vi "next chunk - read-write freq PID file -analysis.vi"(4 "frequency":dbl, 6 "temperature":dbl format="%#_8g", 7 "PID action":T2, 8 "freq PID file OUT":string="peak_PID_scratch.dat", 9 "freq PID file IN":string="peak_PID.dat", 10 "PID freq IN":dbl[](array[numeric]), 11 "sweep folder path":path) -> (0 "temperatures":dbl[](array[numeric]), 1 "frequencies":dbl[][](array[numeric]), 2 "PID freq":dbl[](array[numeric]), 3 "sweep folder path out":path)   [LabVIEW 2012]
uses:
  next chunk read-write PID -- action.ctl
  ctl -- name dispatcher -- action.ctl
  file -- 9w path.vi
  array -- find index - real.vi
  array -- interpolate -- i.vi
  ctl -- name dispatcher.vi
  Q -- check range -- i -- real.vi
  Q - not nan -- real.vi
  <vilib>/Utility/libraryn.llb/Check if File or Folder Exists.vi
  file -- read list of lines.vi
  parse -- find first line.vi
  parse -- get list of matches -- numbers.vi
  <vilib>/Utility/file.llb/Write To Spreadsheet File.vi
  <vilib>/Utility/file.llb/Write To Spreadsheet File (string).vi
panel:
  in  "ctl kind IN":T1
  in  "ctl kind OUT":T1
  out "header":string[](array[string])
  out "number":i32=9
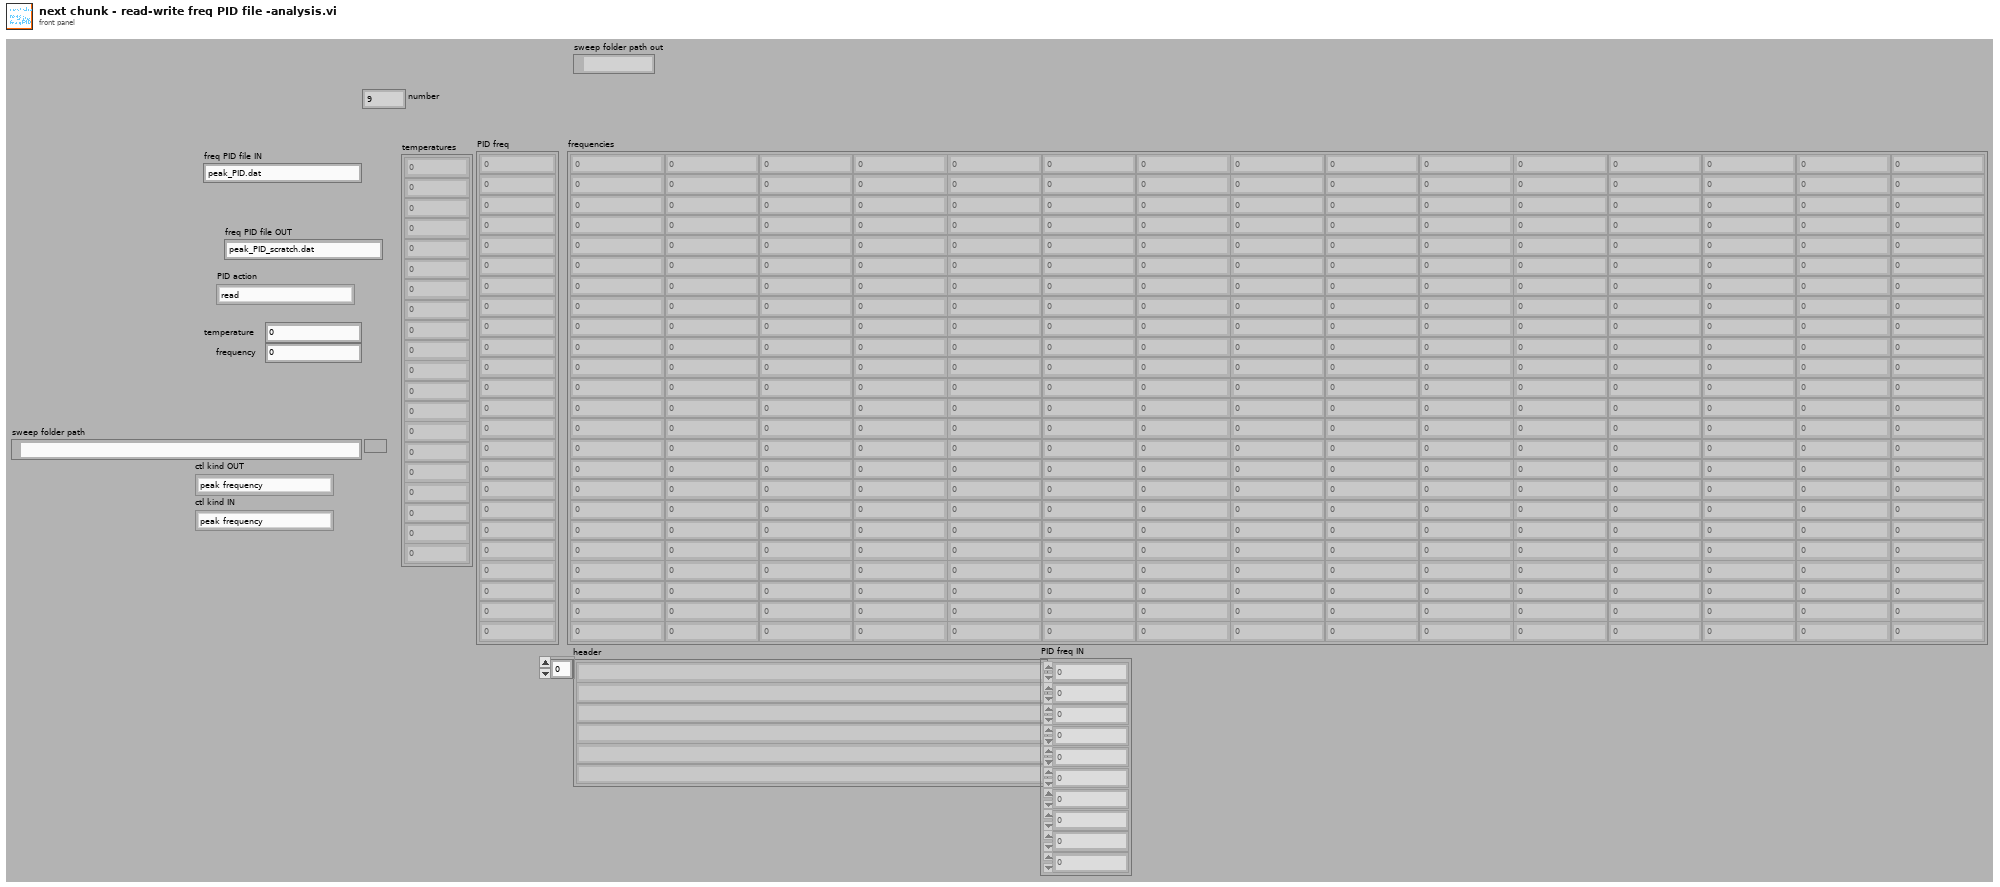
[diagram p1: front panel]
types:
  T1 = typedef "ctl -- name dispatcher -- action.ctl" = enum16{"peak frequency", "peak frequency DUMP", "peak gamma DUMP", "peak gamma", "peak frequency TEST", "peak gamma TEST", "ultrasonic power", "time in gamma", "set temperature ", "set temperature timer", "peak default gamma", "last scan file", "peak freq gamma TEST", "peak NAMES", "errors", "P_I_D", "P", "I", "D"}
  T2 = typedef "next chunk read-write PID -- action.ctl" = enum16{"read", "interpolate", "append col", "write", "write PID col", "append PID col", "interpolate - bezier"}
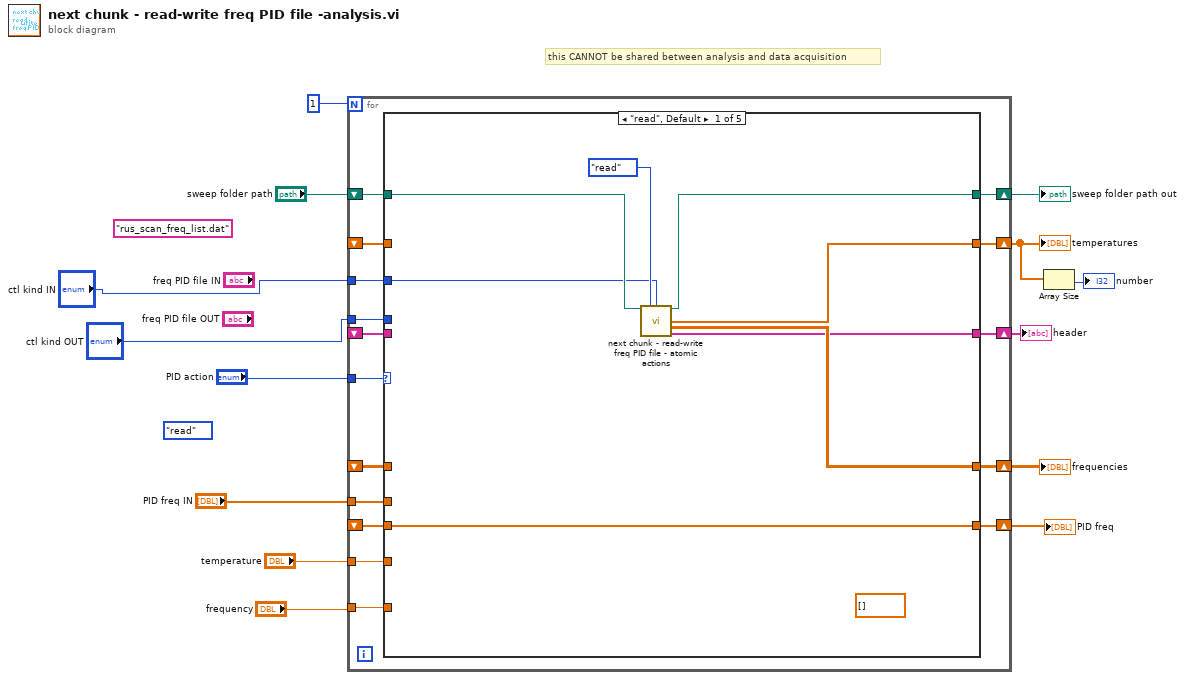
[diagram p0: block diagram]
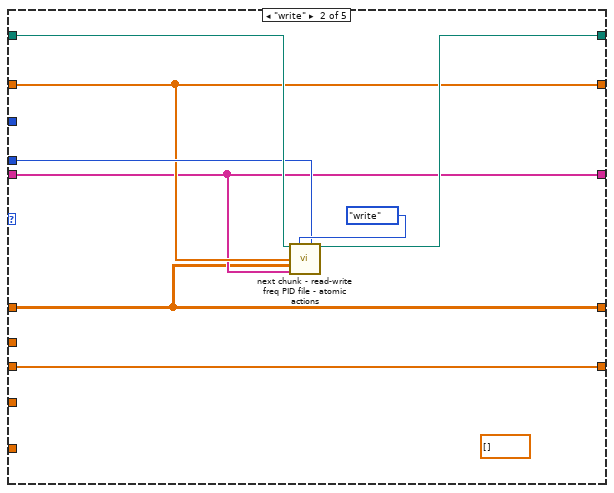
[diagram p2: hidden frame]
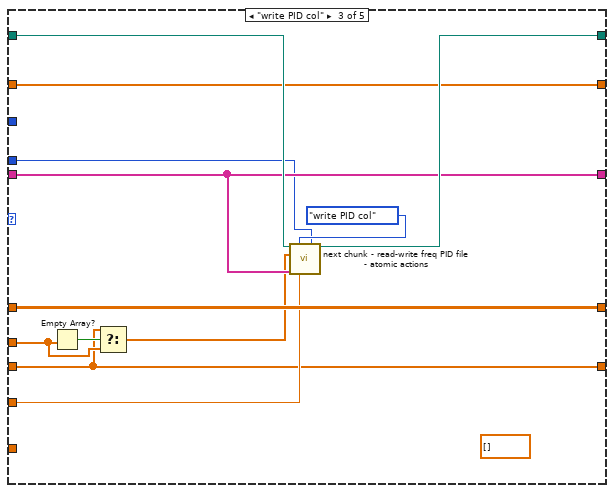
[diagram p3: hidden frame]
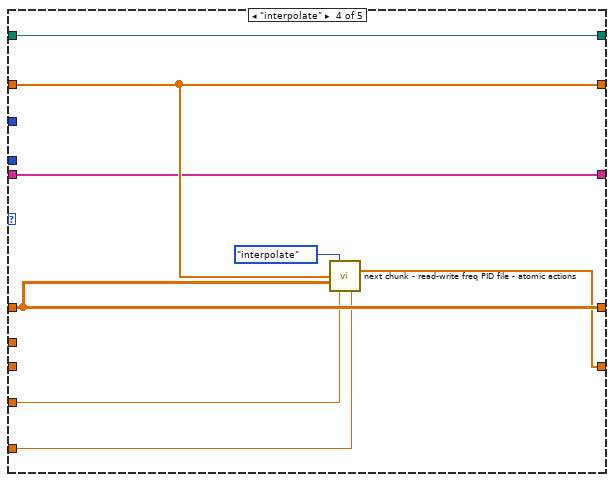
[diagram p4: hidden frame]
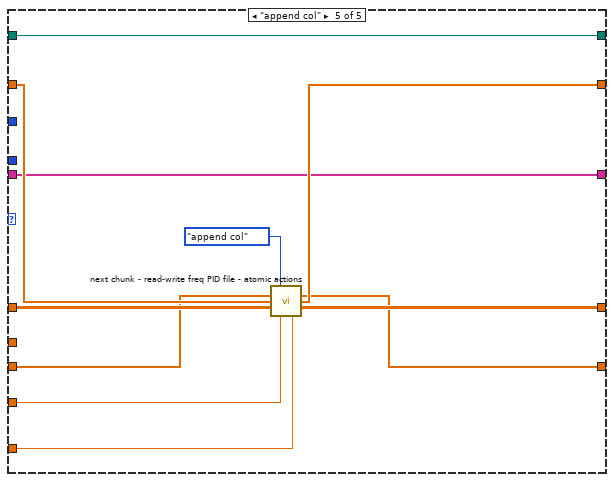
[diagram p5: hidden frame]
diagram:
  (unwired) next_chunk_read-write_PID_--_action."read" ("PID action")
  (unwired) "rus_scan_freq_list.dat" ("delimiter (\\t)")
  # "this CANNOT be shared between analysis and data acquisition"
  n1 = for {
    N: 1 -> [_]
    tunnel: "temperature" -> [w29]
    tunnel: "ctl kind IN" -> [w26]
    tunnel: "PID action" -> [w24]
    shift-right: [w30] -> w5
    shift-left: _ -> [w22]
    shift-right: [w25] -> w9
    shift-left: _ -> [w23]
    shift-right: [w28] -> w13
    shift-left: _ -> [w21]
    tunnel: "ctl kind OUT" -> [w20]
    tunnel: "frequency" -> [w19]
    shift-right: [w18] -> w6
    shift-left: "sweep folder path" -> [w27]
    shift-right: [w17] -> w4
    shift-left: _ -> [w16]
    tunnel: "PID freq IN" -> [w15]
    n2 = case shown="\"read\", Default" w24 {
      tunnel: [w34 w39 w53 w63 w73] -> w30
      tunnel: w29 -> [_ _ w52 w61 w71]
      tunnel: [w38 w46 w49 w62 w67] -> w28
      tunnel: w27 -> [w37 w45 w58 w66 w77]
      tunnel: w26 -> [w32 _ _ _ _]
      tunnel: [w33 w41 w55 w64 w72] -> w25
      tunnel: w23 -> [_ w41 w55 w64 w75]
      tunnel: w22 -> [_ w39 w53 w63 w74]
      tunnel: w21 -> [w38 w46 w49 _ w68]
      tunnel: w20 -> [_ w42 w47 _ _]
      tunnel: w19 -> [_ _ _ w60 w70]
      tunnel: [w36 w44 w57 w66 w77] -> w18
      tunnel: [w31 w40 w54 w59 w69] -> w17
      tunnel: w16 -> [_ w40 w54 w59 w69]
      tunnel: w15 -> [_ _ w50 _ _]
      frame "read", Default {
        (unwired) dbl[] []
        n3 = call "next chunk - read-write freq PID file - atomic actions .vi"("sweep folder path"=w37, "PID action"=next_chunk_read-write_PID_--_action."read", "ctl kind IN"=w32) -> ("sweep folder path out"=w36:path, "temperatures"=w33:dbl[], "frequencies"=w34:dbl[][], "header"=w31:string[])  [unwired: 8 in, 1 out]
      }
      frame "write" {
        (unwired) dbl[] []
        n4 = call "next chunk - read-write freq PID file - atomic actions .vi"("sweep folder path"=w45, "PID action"=next_chunk_read-write_PID_--_action."write", "ctl kind OUT"=w42, "temperatures IN"=w41, "frequencies IN"=w39, "header IN"=w40) -> ("sweep folder path out"=w44:path)  [unwired: 5 in, 4 out]
      }
      frame "write PID col" {
        (unwired) dbl[] []
        n5 = Empty Array?(array=w50) -> (empty?=w51:bool)
        n6 = Select(t=w49, s=w51, f=w50) -> (s? t:f=w48:dbl[])
        n7 = call "next chunk - read-write freq PID file - atomic actions .vi"("sweep folder path"=w58, "PID action"=next_chunk_read-write_PID_--_action."write PID col", "ctl kind OUT"=w47, "PID freq IN"=w48, "header IN"=w54, "temperature"=w52) -> ("sweep folder path out"=w57:path)  [unwired: 5 in, 4 out]
      }
      frame "interpolate" {
        n8 = call "next chunk - read-write freq PID file - atomic actions .vi"("PID action"=next_chunk_read-write_PID_--_action."interpolate", "temperatures IN"=w64, "frequencies IN"=w63, "temperature"=w61, "frequency"=w60) -> ("PID freq"=w62:dbl[])  [unwired: 6 in, 4 out]
      }
      frame "append col" {
        n9 = call "next chunk - read-write freq PID file - atomic actions .vi"("PID action"=next_chunk_read-write_PID_--_action."append col", "PID freq IN"=w68, "temperatures IN"=w75, "frequencies IN"=w74, "temperature"=w71, "frequency"=w70) -> ("PID freq"=w67:dbl[], "temperatures"=w72:dbl[], "frequencies"=w73:dbl[][])  [unwired: 5 in, 2 out]
      }
    }
  }
  "frequencies" <- w5
  "temperatures" <- w9
  "PID freq" <- w13
  "sweep folder path out" <- w6
  "header" <- w4
  n10 = Array Size(array=w9) -> (size(s)=→"number":i32)
